vi "Periodic Tasks.vi"(8 "error in (no error)":errorcluster, 11 "Instance":u32) -> ()   [LabVIEW 2019]
doc: "This VI runs in parallel to other tasks. It can contain as many user-defined periodic loops as you need. These can carry out PID or other sorts of timed response."
uses:
  <vilib>/Rock Robotics/Network Tables/NT Write Number.vi
  <vilib>/Rock Robotics/Network Tables/NT Write Boolean Array.vi
  <vilib>/Rock Robotics/Network Tables/NT Write String Array.vi
  <vilib>/Rock Robotics/Network Tables/NT Globals.vi
  <vilib>/Rock Robotics/Network Tables/NT Write Boolean.vi
  <vilib>/Rock Robotics/Network Tables/NT Write String.vi
  <vilib>/NI_Real-Time Target Support.lvlib
panel:
  out "Client0Too":bool=TRUE
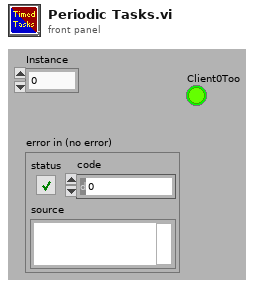
[diagram p1: front panel]
types:
  T1 = enum16{"Add Cnx", "Remove Cnx", "Retrieve List", "Cnx Inited"}
  T2 = typedef "NI_Real-Time Target Support.lvlib/RT CPU Load.ctl" = cluster{"Total (%)":dbl, "Time Critical (%)":dbl, "Timed Structures (%)":dbl, "High (%)":dbl, "Above Normal (%)":dbl, "Normal (%)":dbl, "Background (%)":dbl, "Idle (%)":dbl, "ISR (%)":dbl}
  T3 = typedef "ClientNTTestConfig.ctl" = cluster{"Elapsed0":string, "Name0":string, "Test0":u32, "Ellapsed1":string, "Name1":string, "Test1":u32, "Elapsed2":string, "Name2":string, "Test2":u32, "Elapsed3":string, "Name3":string, "Test3":u32}
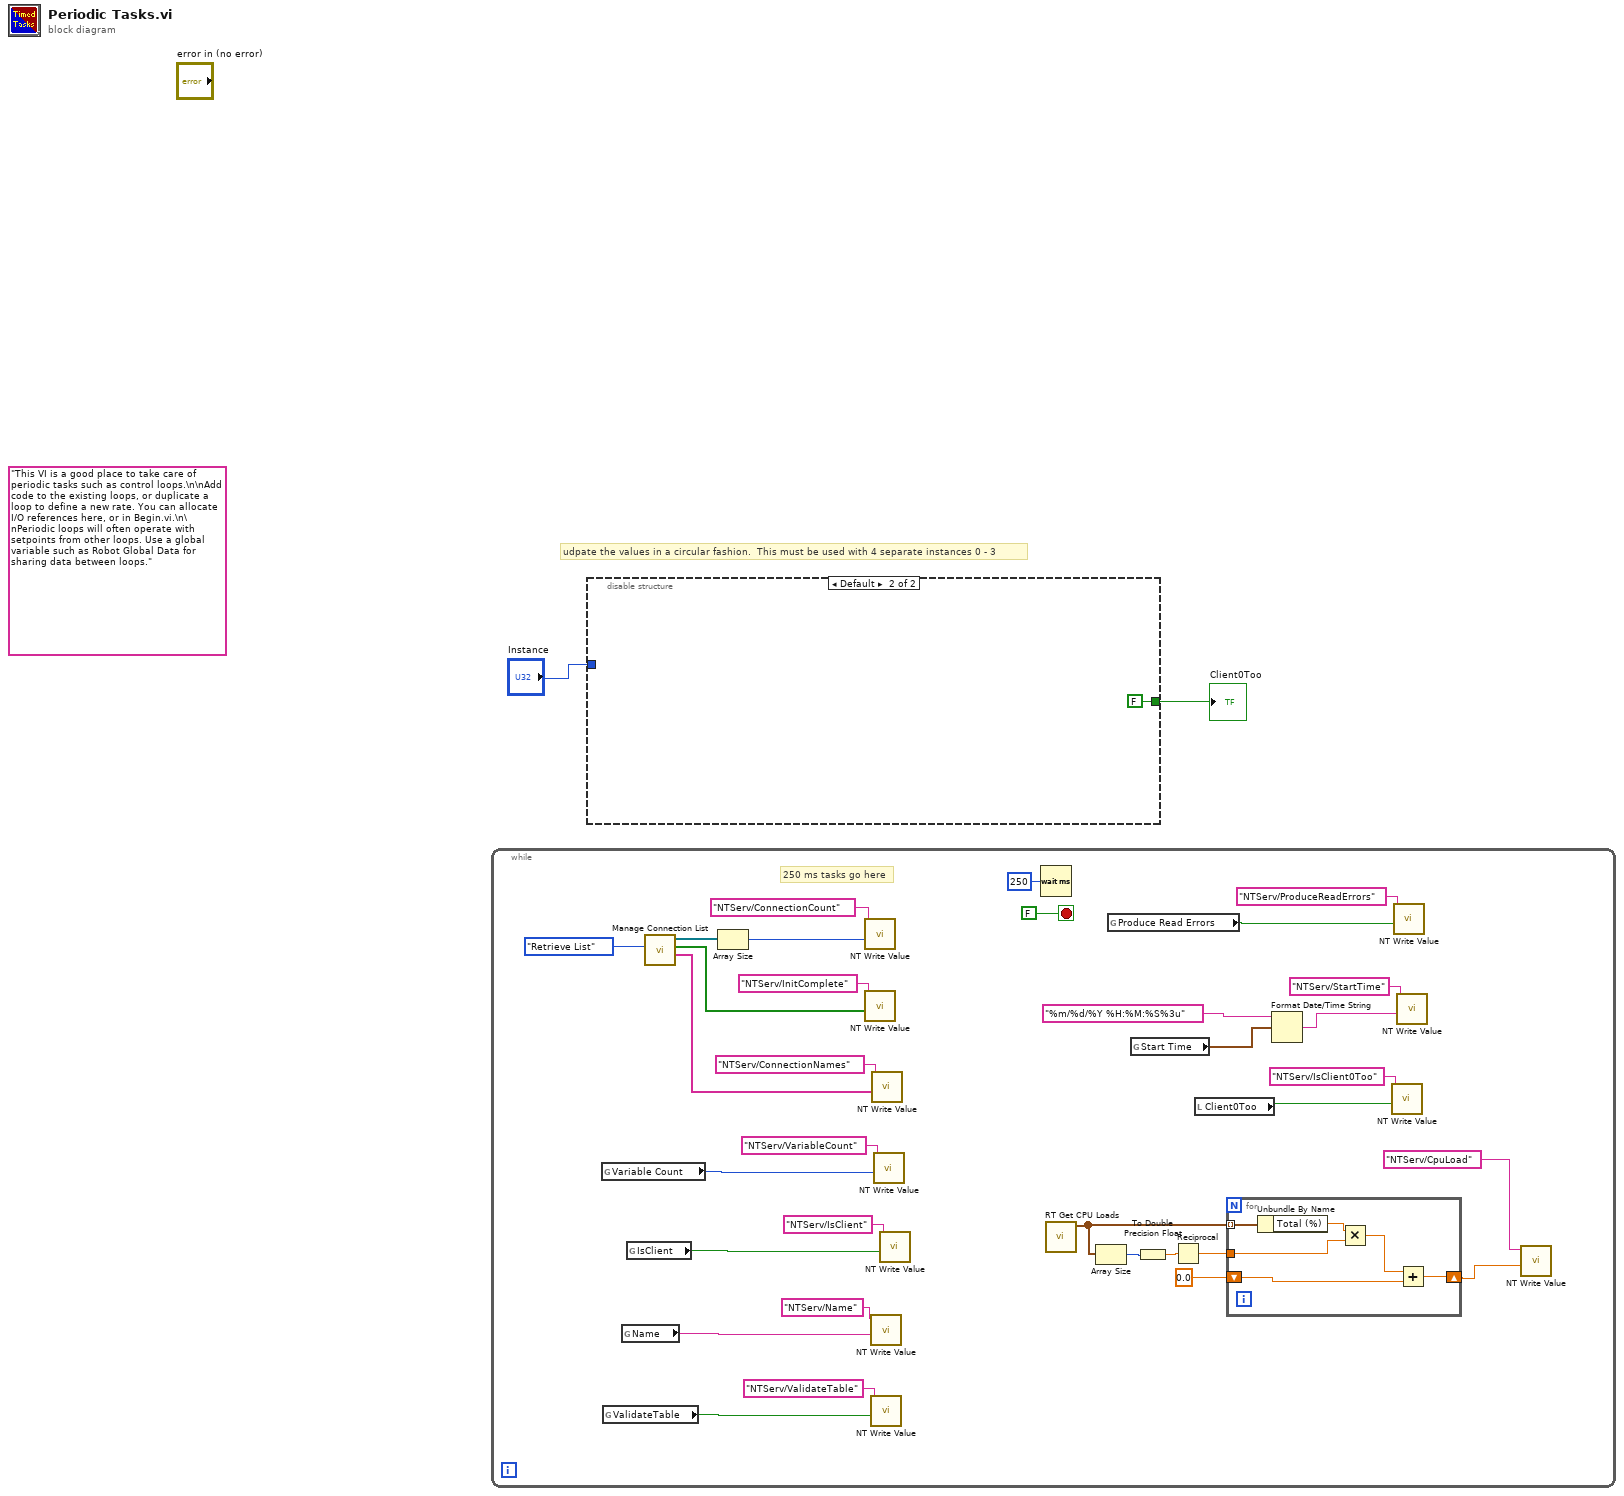
[diagram p0: block diagram]
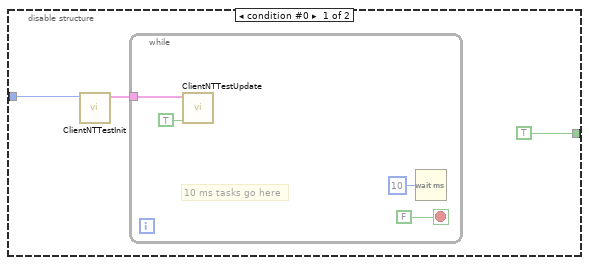
[diagram p2: hidden frame]
diagram:
  (unwired) "This VI is a good place to take care of periodic tasks such as control loops.\n\nAdd code to the existing loops, or duplicate a loop to define a new rate. You can allocate I/O references here, or in Begin.vi.\n\nPeriodic loops will often operate with setpoints from other loops. Use a global variable such as Robot Global Data for sharing data between loops."
  # "udpate the values in a circular fashion.  This must be used with 4 separate instances 0 - 3"
  n1 = while {
    stop <- FALSE stop-if-true
    # "250 ms tasks go here"
    n2 = global read "NT Globals.vi" "Variable Count"() -> (w24:i32)
    n3 = global read "NT Globals.vi" "ValidateTable"() -> (w20:bool)
    n4 = global read "NT Globals.vi" "Name"() -> (w21:string)
    n5 = global read "NT Globals.vi" "IsClient"() -> (w22:bool)
    n6 = call <vilib>:"Manage Connection List.vi"("Operation"=T1."Retrieve List") -> ("Names"=w26:string[], "Inited"=w27:bool[], "Connections List"=w33:refnum<k5>[])  [unwired: 8 in]
    n7 = Array Size(array=w33) -> (size(s)=w31:i32)
    n8 = call-poly <vilib>:"NT Write Value.vi"("Numeric"=w31, "Name"="NTServ/ConnectionCount") -> ()  [unwired: 9 in, 1 out]
    n9 = call-poly <vilib>:"NT Write Value.vi"("Boolean Array"=w27, "Name"="NTServ/InitComplete") -> ()  [unwired: 9 in, 1 out]
    n10 = call-poly <vilib>:"NT Write Value.vi"("String"=w21, "Name"="NTServ/Name") -> ()  [unwired: 9 in, 1 out]
    n11 = call-poly <vilib>:"NT Write Value.vi"("Boolean"=w20, "Name"="NTServ/ValidateTable") -> ()  [unwired: 9 in, 1 out]
    n12 = call-poly <vilib>:"NT Write Value.vi"("String Array"=w26, "Name"="NTServ/ConnectionNames") -> ()  [unwired: 9 in, 1 out]
    n13 = call-poly <vilib>:"NT Write Value.vi"("Numeric"=w24, "Name"="NTServ/VariableCount") -> ()  [unwired: 9 in, 1 out]
    n14 = call-poly <vilib>:"NT Write Value.vi"("Boolean"=w22, "Name"="NTServ/IsClient") -> ()  [unwired: 9 in, 1 out]
    n15 = Wait (ms)(milliseconds to wait=u32 250) -> ()  [unwired: 1 out]
    n16 = call <vilib>:"RT Get CPU Loads.vi"() -> ("CPU loads"=w10:T2[])  [unwired: 10 in, 1 out]
    n17 = Array Size(array=w10) -> (size(s)=w9:i32)
    n18 = global read "NT Globals.vi" "Produce Read Errors"() -> (w17:bool)
    n19 = global read "NT Globals.vi" "Start Time"() -> (w14:timestamp)
    n20 = To Double Precision Float(number=w9) -> (double precision float=w8:dbl)
    n21 = Reciprocal(x=w8) -> (1/x=w7:dbl)
    n22 = local read "Client0Too"() -> (w5:bool)
    n23 = for {
      tunnel: w10 -> [w41] mode=indexing
      tunnel: w7 -> [w39]
      shift-right: [w36] -> w3
      shift-left: 0.0 -> [w38]
      n24 = Unbundle By Name(w41) -> ("Total (%)"=w40:dbl)
      n25 = Multiply(x=w40, y=w39) -> (x*y=w37:dbl)
      n26 = Add(x=w37, y=w38) -> (x+y=w36:dbl)
    }
    n27 = Format Date/Time String(time format string (%c)="%m/%d/%Y %H:%M:%S%3u", seconds (now)=w14) -> (date/time string=w12:string)  [unwired: 1 in]
    n28 = call-poly <vilib>:"NT Write Value.vi"("Boolean"=w5, "Name"="NTServ/IsClient0Too") -> ()  [unwired: 9 in, 1 out]
    n29 = call-poly <vilib>:"NT Write Value.vi"("Boolean"=w17, "Name"="NTServ/ProduceReadErrors") -> ()  [unwired: 9 in, 1 out]
    n30 = call-poly <vilib>:"NT Write Value.vi"("String"=w12, "Name"="NTServ/StartTime") -> ()  [unwired: 9 in, 1 out]
    n31 = call-poly <vilib>:"NT Write Value.vi"("Numeric"=w3, "Name"="NTServ/CpuLoad") -> ()  [unwired: 9 in, 1 out]
  }
  n32 = disable-structure shown="Default" {
    disable-tunnel: "Instance" -> [w43 _]
    disable-tunnel: [TRUE FALSE] -> w1
    frame condition #0 {
      n33 = call "ClientNTTestInit.vi"("Instance"=w43) -> ("TestConfig"=w44:T3)  [unwired: 10 in]
      n34 = while {
        tunnel: w44 -> [w46]
        stop <- FALSE stop-if-true
        # "10 ms tasks go here"
        n35 = call "ClientNTTestUpdate.vi"("NT Connection"=TRUE, "TestConfig"=w46) -> ()  [unwired: 2 in, 8 out]
        n36 = Wait (ms)(milliseconds to wait=u32 10) -> ()  [unwired: 1 out]
      }
    }
    frame condition #1 (active) {
    }
  }
  "Client0Too" <- w1
